vi "GeneratePlayerTrajectory.vi"(10 "InitialPlayerPosition":T2, 11 "PlayerMoves":T3[](array[typedef])) -> (3 "PlayerTrajectory":T1[](array[typedef]))   [LabVIEW 2015, in "TronviewPresentation.lvlib" / "BoardDisplay.lvclass"]
uses:
  BoardDisplay.lvclass
  TronVIEWBotAPI/MovementDirection.ctl
  TronviewGame/Board/Position.ctl
  PlayerTrajectory.ctl
  TronVIEWGameUtilities/TronVIEWGameUtilities.lvlib
  TronviewGame/Board/Board.lvclass
  TronVIEWBotAPI/TronVIEWBotAPI.lvlib
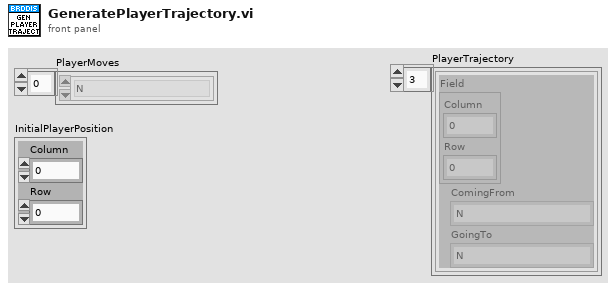
[diagram p1: front panel]
types:
  T1 = typedef "TronviewPresentation.lvlib/BoardDisplay.lvclass/PlayerTrajectory.ctl" = cluster{"Field":T2, "ComingFrom":T3, "GoingTo":T3}
  T2 = typedef "TronviewGame.lvlib/Board.lvclass/Position.ctl" = cluster{"Column":i32, "Row":i32}
  T3 = typedef "TronVIEWBotAPI.lvlib/MovementDirection.ctl" = enum16{"N", "S", "W", "E"}
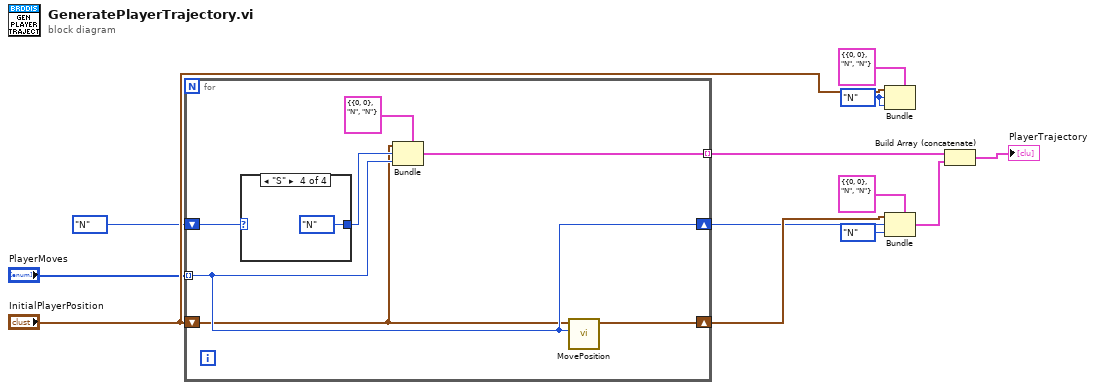
[diagram p0: block diagram]
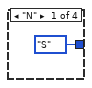
[diagram p2: hidden frame]
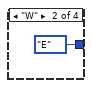
[diagram p3: hidden frame]
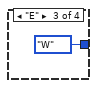
[diagram p4: hidden frame]
diagram:
  w1 = MovementDirection."N" ("ComingFrom")
  n1 = for {
    tunnel: "PlayerMoves" -> [w19] mode=indexing
    shift-right: [w19] -> w7
    shift-left: MovementDirection."N" ("Direction") -> [w16]
    shift-right: [w14] -> w8
    shift-left: "InitialPlayerPosition" -> [w13]
    tunnel: [w17] -> w12 mode=indexing
    n2 = case shown="\"S\"" w16 {
      tunnel: [MovementDirection."S" ("Direction") MovementDirection."E" ("Direction") MovementDirection."W" ("Direction") MovementDirection."N" ("Direction")] -> w15
      frame "N" {
      }
      frame "W" {
      }
      frame "E" {
      }
      frame "S" {
      }
    }
    n3 = Bundle(cluster=T1 {"Field"={"Column"=0, "Row"=0}, "ComingFrom"=enum."N", "GoingTo"=enum."N"} ("TrajectoryField"), "Field"=w13, "ComingFrom"=w15, "GoingTo"=w19) -> (w17:T1)
    n4 = call "MovePosition.vi"("Direction"=w19, "PlayerPosition"=w13) -> ("NewPlayerPosition"=w14:T2)  [unwired: 9 in]
  }
  n5 = Bundle(cluster=T1 {"Field"={"Column"=0, "Row"=0}, "ComingFrom"=enum."N", "GoingTo"=enum."N"} ("TrajectoryField"), "Field"="InitialPlayerPosition", "ComingFrom"=w1, "GoingTo"=w1) -> ()  [unwired: 1 out]
  n6 = Bundle(cluster=T1 {"Field"={"Column"=0, "Row"=0}, "ComingFrom"=enum."N", "GoingTo"=enum."N"} ("TrajectoryField"), "Field"=w8, "ComingFrom"=w7, "GoingTo"=MovementDirection."N") -> (w9:T1)
  n7 = Build Array (concatenate)(w12, w9) -> (→"PlayerTrajectory":T1[])
